vi "SetOccurrence2.vi"(11 "lua_state *L":u64) -> (3 "return":i32=1)   [LabVIEW 2011]
uses:
  lua-5.2.1/src/lua52.dll
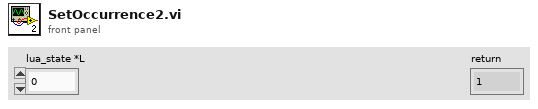
[diagram p1: front panel]
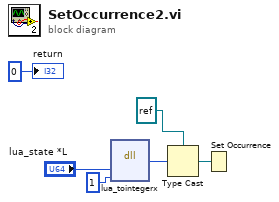
[diagram p0: block diagram]
diagram:
  n1 = dll-call lib="G:/work/LuaDllToLabview/lua-5.2.1/src/lua52.dll" fn="lua_tointegerx"("lua_state *L"="lua_state *L", "index"=1) -> ("tointerger"=w2:i32)  [unwired: 5 in, 2 out]
  n2 = Type Cast(type=refnum<k4> refnum ("事件发生"), x=w2) -> (*(type *) &x=w5:refnum<k4>)
  n3 = Set Occurrence(w5) -> ()
  "return" <- 0 ("index")
